vi "niusrprios Construct Channels.vi"(0 "channel configurations":T1(array[cluster]) {"channel configuration"."frequency" format="%#.3pHz"; "channel configuration"."lo frequency" format="%#.3pHz"; "channel configuration"."level" format="%#_gdBm"}, 1 "scope":string(combo)) -> (4 "enabled channels":string[](array[string]), 6 "enabled channel configurations":T2(array[cluster]) {"frequency" format="%#.3pHz"; "lo frequency" format="%#.3pHz"; "level" format="%#_gdBm"})   [LabVIEW 2015]
doc: "Constructs arrays of channels and configurations from the <B>scope</B> and <B>channel configurations</B>. For example, if the <B>enabled channels</B> boolean array has elements 0 and 1 both TRUE with a <B>scope</B> of \"rx\", the resulting <B>channels</B> array will be [\"rx/RF 0\", \"rx/RF 1\"]."
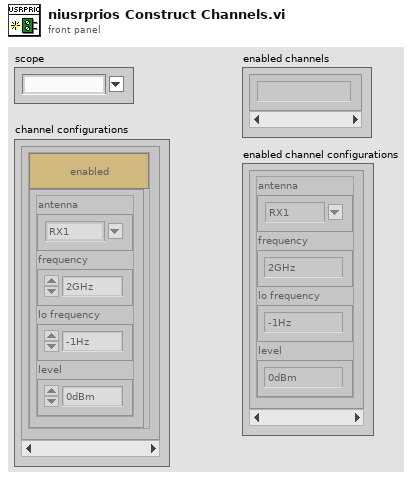
[diagram p1: front panel]
types:
  T1 = cluster{"channel enable":bool, "channel configuration":cluster{"antenna":string, "frequency":dbl, "lo frequency":dbl, "level":dbl}}[]
  T2 = cluster{"antenna":string, "frequency":dbl, "lo frequency":dbl, "level":dbl}[]
  T3 = cluster{"antenna":string, "frequency":dbl, "lo frequency":dbl, "level":dbl}
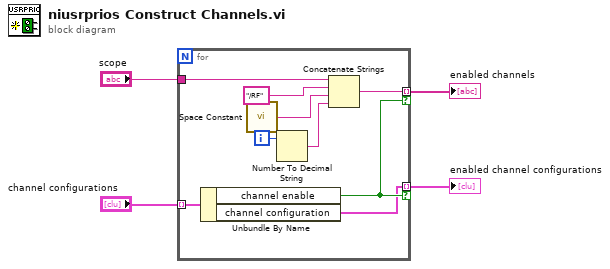
[diagram p0: block diagram]
diagram:
  n1 = for {
    tunnel: "scope" -> [w13]
    tunnel: [w10] -> w4 mode=indexing if=w6
    tunnel: [w5] -> w1 mode=indexing if=w6
    tunnel: "channel configurations" -> [w7] mode=indexing
    i -> [w11]
    n2 = Unbundle By Name(w7) -> ("channel enable"=w6:bool, "channel configuration"=w5:T3)
    n3 = call <vilib>:"Space Constant.vi"() -> ("String"=w8:string)
    n4 = Number To Decimal String(number=w11) -> (decimal integer string=w12:string)  [unwired: 1 in]
    n5 = Concatenate Strings(w13, "/RF" ("string"), w8, w12) -> (w10:string)
  }
  "enabled channels" <- w4
  "enabled channel configurations" <- w1
